vi "Change sign B _X if necessary (SubVI).vi"(10 "Magnetic field x [µT] in":dbl, 11 "Octant":string) -> (3 "Magnetic field x [µT] out":dbl)   [LabVIEW 2018]
panel:
  # "The actual signals being sent to the PS for certain octant combinations don't change. However, the way the cables are connected have been changed. This means the magnetic field being generated by the coils changes too, which needs to be reflected by the indicators. This is what these blocks of code do: change the sign of the magnetic field strength being displayed on the screen."
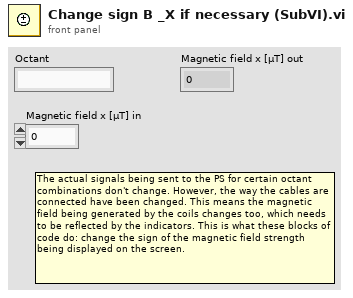
[diagram p1: front panel]
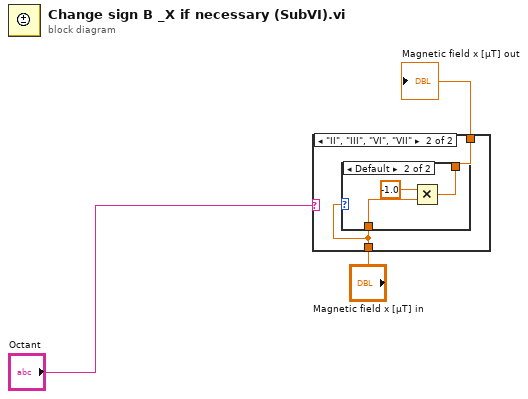
[diagram p0: block diagram]
diagram:
  n1 = case shown="\"II\", \"III\", \"VI\", \"VII\"" "Octant" {
    tunnel: "Magnetic field x [µT] in" -> [w4 w5]
    tunnel: [w4 w6] -> w2
    frame "I", "IV", "V", "VIII", Default {
    }
    frame "II", "III", "VI", "VII" {
      n2 = case shown="Default" w5 {
        tunnel: [w7 w9] -> w6
        tunnel: w5 -> [w7 w8]
        frame 0 {
        }
        frame Default {
          n3 = Multiply(x=-1.0, y=w8) -> (x*y=w9:dbl)
        }
      }
    }
  }
  "Magnetic field x [µT] out" <- w2
